vi "环境参数table定义.vi"(10 "table 输入":string, 11 "data":T1={"时间标识"=timestamp(0 s since 1904-01-01), "测量模式"="水样测试", "数据类型"="N", "监测值"=0.0, "单位"="mg/L", "数据标识"="N", "因子编码"=""}) -> (1 "table 输出":string, 2 "columns":string[](array[string]), 3 "data输出":T1={"时间标识"=timestamp(0 s since 1904-01-01), "测量模式"="水样测试", "数据类型"="N", "监测值"=0.0, "单位"="mg/L", "数据标识"="N", "因子编码"=""})   [LabVIEW 2016, in "流量计.lvlib"]
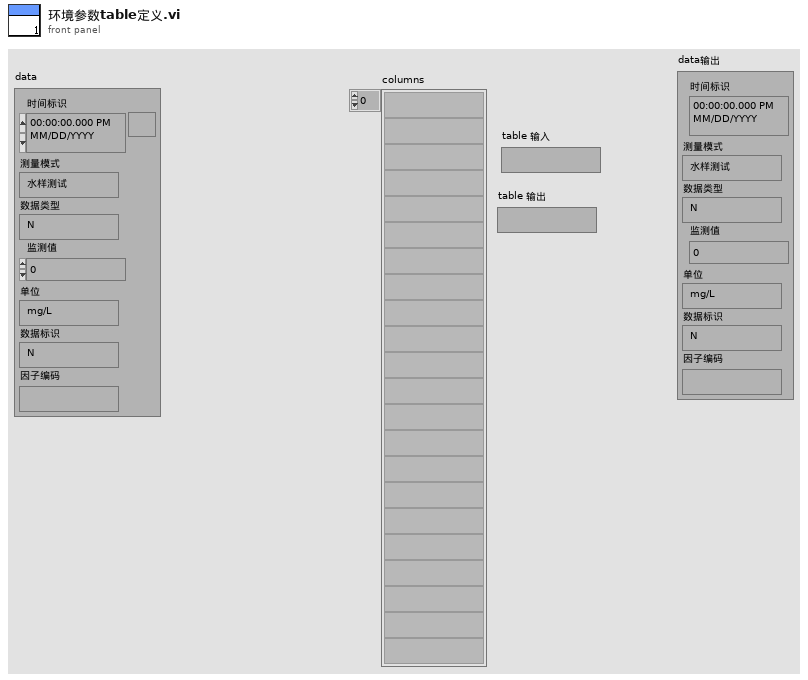
[diagram p1: front panel]
types:
  T1 = cluster{"时间标识":timestamp, "测量模式":string, "数据类型":string, "监测值":sgl, "单位":string, "数据标识":string, "因子编码":string}
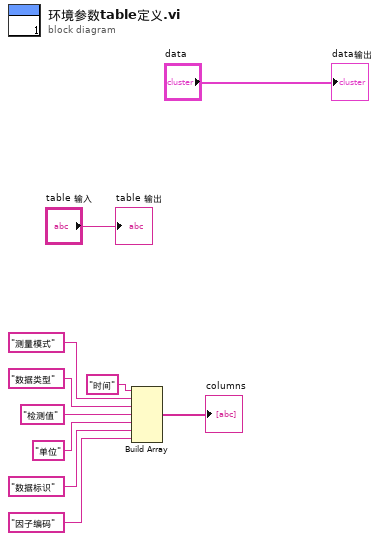
[diagram p0: block diagram]
diagram:
  n1 = Build Array("时间", "测量模式", "数据类型", "检测值", "单位", "数据标识", "因子编码") -> (→"columns":string[])
  "table 输出" <- "table 输入"
  "data输出" <- "data"
